vi "Validate Source Parameters.vi"(8 "error in (no error)":errorcluster, 11 "measurement configuration":T1={"Mode of operation"=enum."Perform measurement", "DUT setup time"=1.0, "Source delay"=0.005, "Aperture time"=0.005, "Nominal output voltage"=3.3, "Source pin name array"=[], "Source pin name index for efficiency"=0, "Source sense array"=[], "Source current limit array"=[], "Source maximum power array"=[], "Source start voltage array"=[], "Source stop voltage array"=[], "Source voltage sweep points"=4, "Use Source voltage array"=FALSE, "Source voltage concatenated array"=[], "Source voltage array size"=[], "Load pin name"="", "Load sense"=1009, "Load voltage limit range"=6.0, "Load sweep type"="Logarithmic", "Load start current"=0.1, "Load stop current"=24.0, "Load current sweep points/points per decade"=10, "Use Load current array"=FALSE, "Load current array"=[], "Pin Names for Scope"=[], "vertical range"=[], "vertical offset"=[], "probe attenuation"=[], "vertical coupling"=[], "channel enabled"=[], "input impedance"=[], "max input frequency"=[], "min sample rate"=[], "reference position"=[], "min record length"=[], "enforce realtime"=[], "dmm pin names"=[], "dmm function array"=[], "dmm resolution in digits array"=[], "dmm range array"=[]} {"dmm function array" items=["DC Volts", "AC Volts", "DC Current", "AC Current", "2-wire Resistance", "4-wire Resistance", "Diode", "Frequency", "Period", "AC Volts DC Coupled", "Capacitance", "Inductance", "Temperature"]; "Source sense array" items=["Local"=1008, "Remote"=1009]; "dmm resolution in digits array" items=["3 1/2"=3.5, "4 1/2"=4.5, "5 1/2"=5.5, "6 1/2"=6.5, "7 1/2"=7.5]; "input impedance" items=["1 mega ohm"=0, "50 ohms"=2]; "vertical coupling" items=["AC", "DC", "Ground"]; "Load sense" items=["Local"=1008, "Remote"=1009]}) -> (0 "error out":errorcluster)   [LabVIEW 2021, in "Efficiency And Load Regulation with Pin Map.lvlib"]
uses:
  Efficiency And Load Regulation with Pin Map.lvlib
  Measurement Configuration.ctl
  <instrlib>/niScope/Controls/niScope vertical coupling.ctl
  <instrlib>/niDMM/nidmm.llb/niDMM Resolution in Digits.ctl
  <vilib>/Utility/error.llb/Error Cluster From Error Code.vi
  <vilib>/ErrorRing/Error Ring.xnode
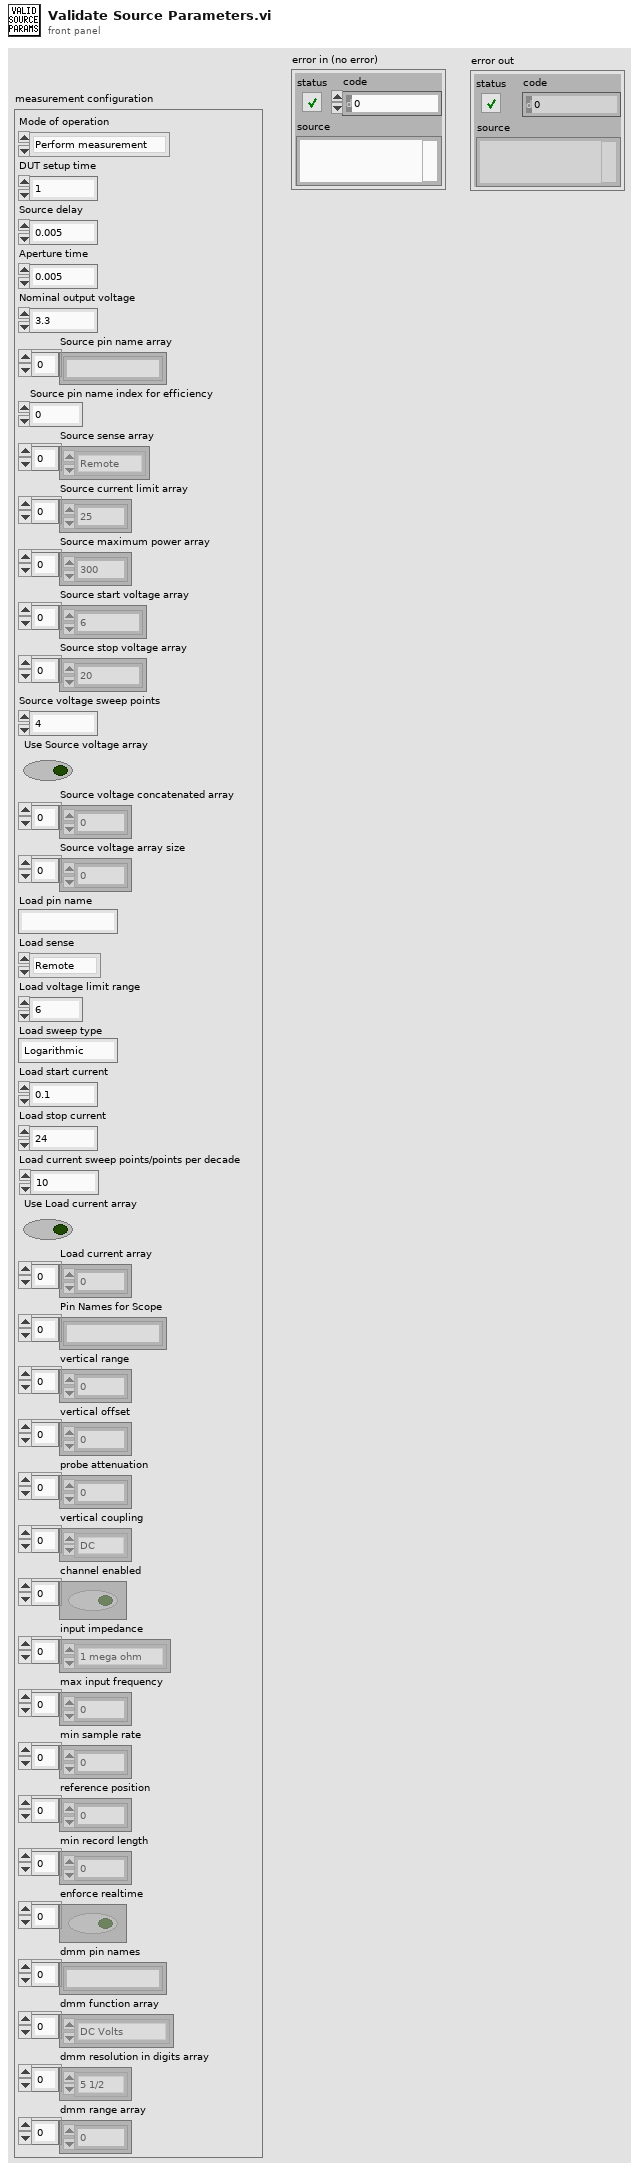
[diagram p1: front panel]
types:
  T1 = typedef "Efficiency And Load Regulation with Pin Map.lvlib/Measurement Configuration.ctl" = cluster{"Mode of operation":enum32{"Power on the DUT", "Perform measurement", "Power off the DUT"}, "DUT setup time":dbl, "Source delay":dbl, "Aperture time":dbl, "Nominal output voltage":dbl, "Source pin name array":string[], "Source pin name index for efficiency":i32, "Source sense array":i32[], "Source current limit array":dbl[], "Source maximum power array":dbl[], "Source start voltage array":dbl[], "Source stop voltage array":dbl[], "Source voltage sweep points":i32, "Use Source voltage array":bool, "Source voltage concatenated array":dbl[], "Source voltage array size":i32[], "Load pin name":string, "Load sense":i32, "Load voltage limit range":dbl, "Load sweep type":string, "Load start current":dbl, "Load stop current":dbl, "Load current sweep points/points per decade":i32, "Use Load current array":bool, "Load current array":dbl[], "Pin Names for Scope":string[], "vertical range":dbl[], "vertical offset":dbl[], "probe attenuation":dbl[], "vertical coupling":T2[], "channel enabled":bool[], "input impedance":u32[], "max input frequency":dbl[], "min sample rate":dbl[], "reference position":dbl[], "min record length":i32[], "enforce realtime":bool[], "dmm pin names":string[], "dmm function array":u32[], "dmm resolution in digits array":T3[], "dmm range array":dbl[]}
  T2 = typedef "niScope vertical coupling.ctl" = i32
  T3 = typedef "niDMM Resolution in Digits.ctl" = dbl
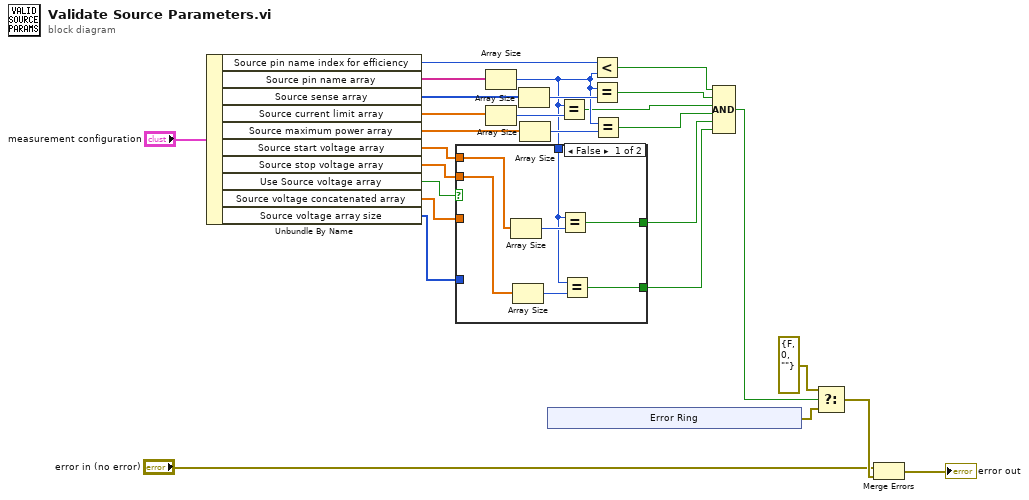
[diagram p0: block diagram]
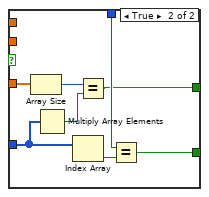
[diagram p2: hidden frame]
diagram:
  n1 = Unbundle By Name("measurement configuration") -> ("Source pin name index for efficiency"=w19:i32, "Source pin name array"=w26:string[], "Source sense array"=w21:i32[], "Source current limit array"=w25:dbl[], "Source maximum power array"=w24:dbl[], "Source start voltage array"=w2:dbl[], "Source stop voltage array"=w1:dbl[], "Use Source voltage array"=w15:bool, "Source voltage concatenated array"=w16:dbl[], "Source voltage array size"=w18:i32[])
  n2 = Array Size(array=w26) -> (size(s)=w17:i32)
  n3 = case shown="False" w15 {
    tunnel: w18 -> [_ w39]
    tunnel: w17 -> [w30 w41]
    tunnel: w16 -> [_ w40]
    tunnel: [w33 w36] -> w10
    tunnel: [w31 w35] -> w9
    tunnel: w2 -> [w29 _]
    tunnel: w1 -> [w28 _]
    frame False {
      n4 = Array Size(array=w29) -> (size(s)=w34:i32)
      n5 = Array Size(array=w28) -> (size(s)=w32:i32)
      n6 = Equal?(x=w30, y=w34) -> (x = y?=w33:bool)
      n7 = Equal?(x=w30, y=w32) -> (x = y?=w31:bool)
    }
    frame True {
      n8 = Array Size(array=w40) -> (size(s)=w38:i32)
      n9 = Multiply Array Elements(1:w39) -> (0:w37:i32)
      n10 = Index Array(array=w39) -> (element=w42:i32)  [unwired: 1 in]
      n11 = Equal?(x=w38, y=w37) -> (x = y?=w36:bool)
      n12 = Equal?(x=w41, y=w42) -> (x = y?=w35:bool)
    }
  }
  n13 = Array Size(array=w25) -> (size(s)=w22:i32)
  n14 = Array Size(array=w21) -> (size(s)=w20:i32)
  n15 = Array Size(array=w24) -> (size(s)=w23:i32)
  n16 = xnode "Error Ring"() -> ("error out"=w7:errorcluster)
  n17 = Equal?(x=w17, y=w22) -> (x = y?=w12:bool)
  n18 = Less?(x=w19, y=w17) -> (x < y?=w14:bool)
  n19 = Equal?(x=w17, y=w20) -> (x = y?=w13:bool)
  n20 = Equal?(x=w17, y=w23) -> (x = y?=w11:bool)
  n21 = Compound Arithmetic op=AND(w14, w13, w12, w11, w10, w9) -> (w8:bool)
  n22 = Select(t=errorcluster {"status"=FALSE, "code"=0, "source"=""}, s=w8, f=w7) -> (s? t:f=w5:errorcluster)
  n23 = Merge Errors("error in (no error)", w5) -> (→"error out":errorcluster)
